vi "Write Bit.vi"(8 "error in (no error)":errorcluster caption="error in", 9 "ON/OFF":bool, 10 "Address":u16=65535 format="%.0x", 11 "Port Selection Info In":T1={"Port Name"="", "Amplifier Num"=1, "Baud Rate"=38400, "Char Formation"=enum."0"} {"Baud Rate" items=["38400"=38400, "19200"=19200, "9600"=9600, "115200"=0]; "Amplifier Num" max=31}) -> (0 "error out":errorcluster, 3 "Port Selection Info Out":T1={"Port Name"="", "Amplifier Num"=1, "Baud Rate"=38400, "Char Formation"=enum."0"} {"Baud Rate" items=["38400"=38400, "19200"=19200, "9600"=9600, "115200"=0]; "Amplifier Num" max=31})   [LabVIEW 2014, in "ALPHA5 RS485.lvlib"]
uses:
  ALPHA5 RS485.lvlib
  typedefs/Port Selection Info.ctl
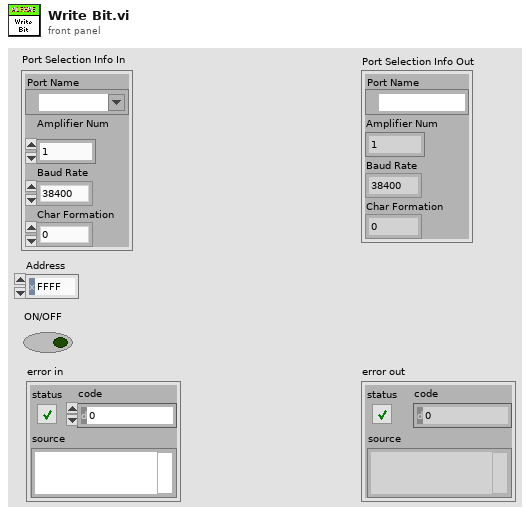
[diagram p1: front panel]
types:
  T1 = typedef "ALPHA5 RS485.lvlib/Port Selection Info.ctl" = cluster{"Port Name":refnum<visa-resource-name>, "Amplifier Num":u8, "Baud Rate":u32, "Char Formation":enum16{"0", "1", "2", "3", "4", "5"}}
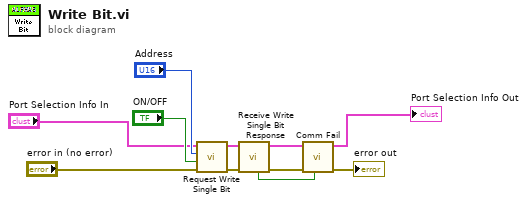
[diagram p0: block diagram]
diagram:
  n1 = call "Request Write Single Bit.vi"("error in (no error)"="error in (no error)", "ON/OFF"="ON/OFF", "Address"="Address", "Port Selection Info"="Port Selection Info In") -> ("error out"=w9:errorcluster, "Port Selection Info Out"=w10:T1)  [unwired: 6 in]
  n2 = call "Receive Write Single Bit Response.vi"("error in (no error)"=w9, "Port Selection Info"=w10) -> ("error out"=w4:errorcluster, "Port Selection Info Out"=→"Port Selection Info Out":T1, "CRC Match"=w1:bool)  [unwired: 3 in, 4 out]
  n3 = call "Comm Fail.vi"("CRC Match"=w1, "error in (no error)"=w4) -> ("error out"=→"error out":errorcluster)  [unwired: 9 in]
